vi "PMBus Set Control.vi"(7 "Value":u8, 8 "error in (no error)":errorcluster, 9 "PMBusIndex":i32, 10 "DevIndex":i32, 11 "DevType":i32) -> (0 "error out":errorcluster, 3 "function return":i32)   [LabVIEW 2012, in "ControlPMBus.lvlib"]
doc: "int WINAPI PMBus_SetControl(int DevType,int DevIndex,int PMBusIndex,unsigned char Value);"
uses:
  ControlPMBus.lvlib
  Ginkgo_Driver.dll
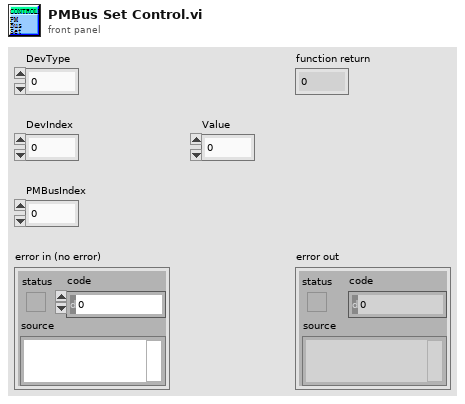
[diagram p1: front panel]
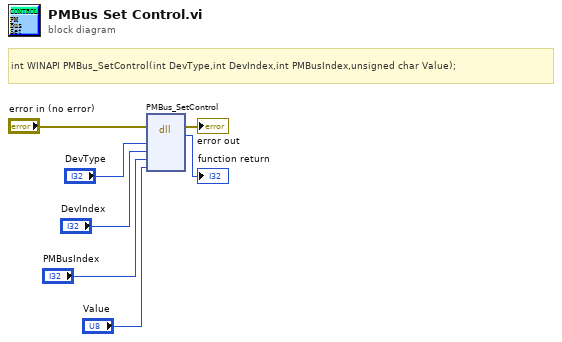
[diagram p0: block diagram]
diagram:
  # "int WINAPI PMBus_SetControl(int DevType,int DevIndex,int PMBusIndex,unsigned char Value);"
  n1 = dll-call lib="E:/Project/vt_ginkgo/truck/Ginkgo Driver/vs2010/Ginkgo_USB-I2C_API_v2.0.3.0/lib/labview_32bit/ControlPMBus/Ginkgo_Driver.*" fn="PMBus_SetControl"(error in="error in (no error)", "DevType"="DevType", "DevIndex"="DevIndex", "PMBusIndex"="PMBusIndex", "Value"="Value") -> (error out=→"error out":errorcluster, →"function return":i32)  [unwired: 6 in, 1 out]
